vi "GD Errors in Status.vi"(6 "get Test Data":bool, 8 "error in (no error)":errorcluster caption="Fehler (Eingang, kein Fehler)", 9 "Sprachliste":string[][](array[string]), 11 "Status in":string caption="Status") -> (0 "error out":errorcluster caption="Fehler (Ausgang)", 3 "Statusout":string caption="Status")   [LabVIEW 2020, in "Linearisierung v2.lvlib"]
uses:
  Linearisierung v2.lvlib
  Aktion FGV Stoerungen sammeln und auswerten.ctl
  SpanEinstellungen/GD Info Cluster.ctl
  LIN ErrorCluster.ctl
  SpanEinstellungen/Aktion FGV Spans abarbeiten.ctl
  Aktion FGV GD Status Anzeige.ctl
  SpanEinstellungen/Aktion FGV GD Errors sammeln.ctl
  SpanEinstellungen/SpanEinstellungen.lvlib
  Gasteiler/Gasteiler.lvlib
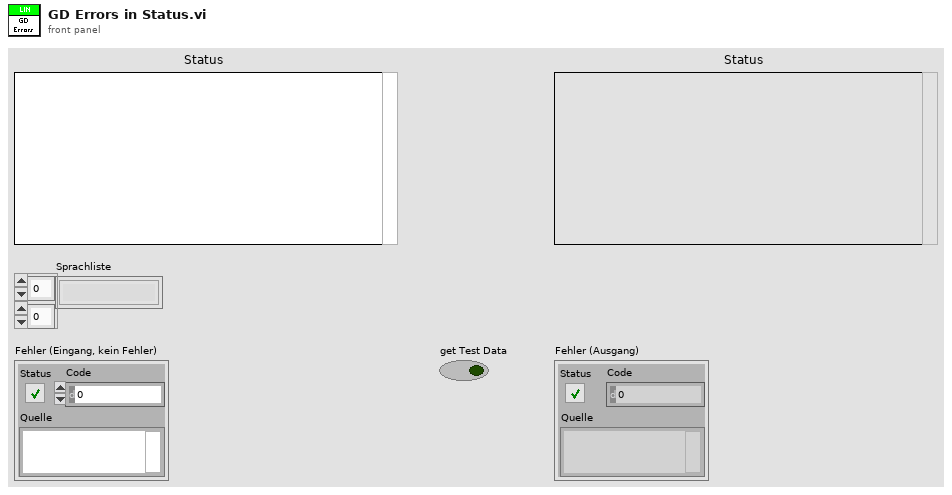
[diagram p1: front panel]
types:
  T1 = typedef "Linearisierung v2.lvlib/Aktion FGV Stoerungen sammeln und auswerten.ctl" = enum16{"init", "lesen", "error", "prüfen", "reset error", "abbrechen", "fortsetzen", "neustart", "Bedientasten reset"}
  T2 = typedef "Linearisierung v2.lvlib/LIN ErrorCluster.ctl" = cluster{"Störung Kommunikation":bool, "Pressure carrier gas":bool, "Pressure diluted gas":bool, "Outlet Pressure":bool, "SNOX before SAIR":bool, "Störung Gasteiler":bool}
  T3 = typedef "Linearisierung v2.lvlib/SpanEinstellungen.lvlib/GD Info Cluster.ctl" = cluster{"Wobei":string, "Status":string, "Errors":T2, "Empfangsdaten":string[], "Zeitstempel":string}
  T4 = typedef "Linearisierung v2.lvlib/Aktion FGV GD Status Anzeige.ctl" = enum16{"lesen", "schreiben", "hinzufügen"}
  T5 = typedef "Linearisierung v2.lvlib/SpanEinstellungen.lvlib/Aktion FGV Spans abarbeiten.ctl" = enum16{"lesen", "idle", "start", "next", "comp", "init", "running", "abort"}
  T6 = typedef "Linearisierung v2.lvlib/SpanEinstellungen.lvlib/Aktion FGV GD Errors sammeln.ctl" = enum16{"lesen", "init", "GD Infos sammeln", "Kalibrierinfos sammeln", "Test Data", "GD Infos selektiv sammeln"}
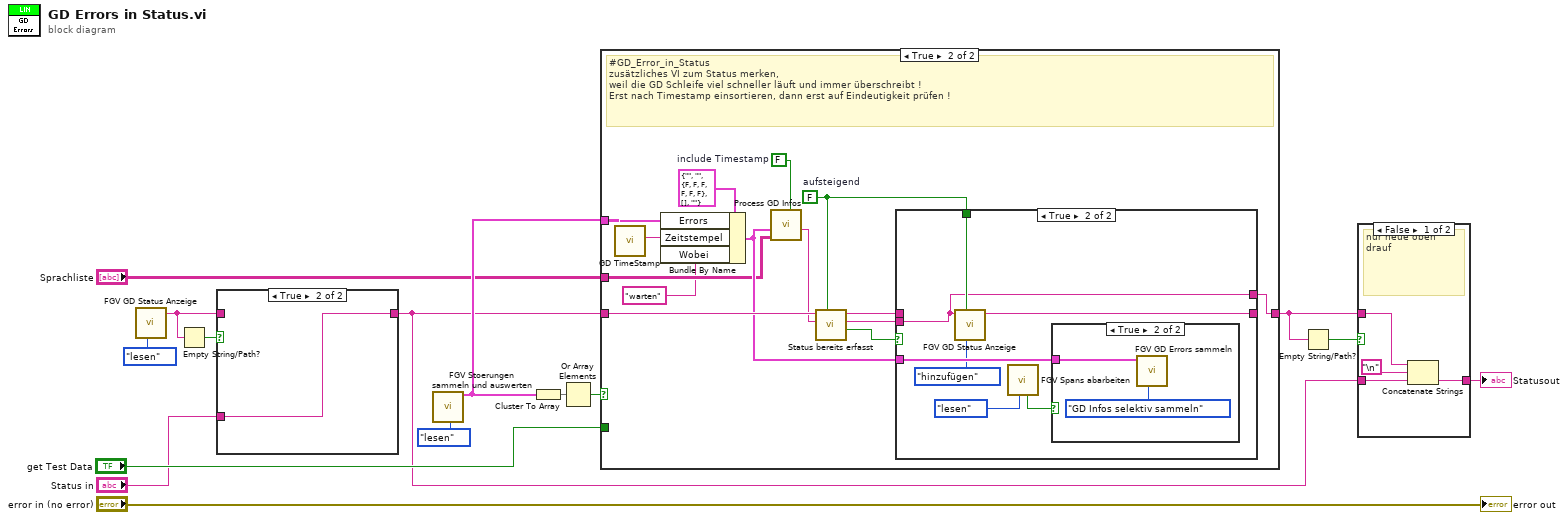
[diagram p0: block diagram]
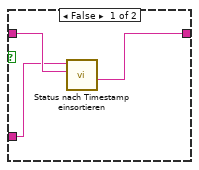
[diagram p2: hidden frame]
diagram:
  n1 = call "FGV GD Status Anzeige.vi"("Aktion"=enum16{"lesen", "schreiben", "hinzufügen"}."lesen") -> ("Zustand out"=w3:string)  [unwired: 9 in, 1 out]
  n2 = Empty String/Path?(string/path=w3) -> (empty?=w4:bool)
  n3 = case shown="True" w4 {
    tunnel: "Status in" -> [w16 w19]
    tunnel: w3 -> [w18 _]
    tunnel: [w17 w19] -> w1
    frame False {
      n4 = call "Status nach Timestamp einsortieren.vi"("GD Statuslist in"=w18, "Statuslist old in"=w16) -> ("merged Statuslist sorted"=w17:string)  [unwired: 6 in, 3 out]
    }
    frame True {
    }
  }
  n5 = call "FGV Stoerungen sammeln und auswerten.vi"("Aktion"=Aktion_FGV_Stoerungen_sammeln_und_auswerten."lesen") -> ("Errors"=w13:T2)  [unwired: 12 in, 6 out]
  n6 = Cluster To Array(cluster=w13) -> (array=w15:bool[])
  n7 = Or Array Elements(Boolean array=w15) -> (logical OR=w12:bool)
  n8 = case shown="True" w12 {
    tunnel: w13 -> [_ w32]
    tunnel: [w20 w21] -> w6
    tunnel: w1 -> [w20 w31]
    tunnel: "Sprachliste" -> [_ w26]
    tunnel: "get Test Data" -> [_ _]
    frame False {
    }
    frame True {
      w25 = FALSE  # aufsteigend
      w28 = FALSE  # include Timestamp
      # "#GD_Error_in_Status\nzusätzliches VI zum Status merken,\nweil die GD Schleife viel schneller läuft und immer überschreibt !\nErst nach Timestamp einsortieren, dann erst auf Eindeutigkeit prüfen !"
      n9 = call "GD TimeStamp.vi"() -> ("date/time string"=w34:string)  [unwired: 10 in, 1 out]
      n10 = Bundle By Name(cluster=T3 {"Wobei"="", "Status"="", "Errors"={"Störung Kommunikation"=FALSE, "Pressure carrier gas"=FALSE, "Pressure diluted gas"=FALSE, "Outlet Pressure"=FALSE, "SNOX before SAIR"=FALSE, "Störung Gasteiler"=FALSE}, "Empfangsdaten"=[], "Zeitstempel"=""} ("GD Info-Cluster in"), "Errors"=w32, "Zeitstempel"=w34, "Wobei"="warten") -> (w27:T3)
      n11 = call "Process GD Infos.vi"("include Timestamp"=w28, "Sprachliste"=w26, "GD Info-Cluster in"=w27) -> ("GD Infos"=w30:string)  [unwired: 6 in, 2 out]
      n12 = call "Status bereits erfasst.vi"("aufsteigend"=w25, "Status new in"=w30, "Status old in"=w31) -> ("unique"=w22:bool, "Status new out"=w24:string, "Status old out"=w29:string)  [unwired: 5 in, 1 out]
      n13 = case shown="True" w22 {
        tunnel: w27 -> [_ w40]
        tunnel: [w35 w37] -> _
        tunnel: w29 -> [w35 _]
        tunnel: w25 -> [_ w38]
        tunnel: w24 -> [_ w36]
        tunnel: [_ w36] -> w21
        frame False {
        }
        frame True {
          n14 = call "FGV GD Status Anzeige.vi"("Aktion"=Aktion_FGV_GD_Status_Anzeige."hinzufügen", "aufsteigend"=w38, "Zustand in"=w36) -> ("Zustand out"=w37:string)  [unwired: 7 in, 1 out]
          n15 = call "FGV Spans abarbeiten.vi"("Aktion"=Aktion_FGV_Spans_abarbeiten."lesen") -> ("running out"=w41:bool)  [unwired: 5 in, 5 out]
          n16 = case shown="True" w41 {
            tunnel: w40 -> [_ w43]
            frame False {
            }
            frame True {
              n17 = call "FGV GD Errors sammeln.vi"("Aktion"=Aktion_FGV_GD_Errors_sammeln."GD Infos selektiv sammeln", "GD Info-Cluster in"=w43) -> ()  [unwired: 7 in, 3 out]
            }
          }
        }
      }
    }
  }
  n18 = Empty String/Path?(string/path=w6) -> (empty?=w8:bool)
  n19 = case shown="False" w8 {
    tunnel: w1 -> [w47 w49]
    tunnel: [w45 w49] -> w7
    tunnel: w6 -> [w48 _]
    frame False {
      # "nur neue oben drauf"
      n20 = Concatenate Strings(w48, "\n", w47) -> (w45:string)
    }
    frame True {
    }
  }
  "Statusout" <- w7
  "error out" <- "error in (no error)"
